vi "ReCalc_V2.00 - Kopie.vi"(3 "Berechnen":bool, 4 "Datenspeicher":T2={"Fahrzeugdaten"="", "date/time string"="", "Rolle [Inkr/U]"=0, "Rollenumfang [m]"=0.0, "Rollenträgheit [kgm²]"=0.0, "Zündung [Imp/U]"=0.0, "Getriebe [1:]"=0.0, "Reifenumfang [m] "=0.0, "element"=0.0, "Gl. Mittelwert"=0, "Differenzenquotient"=0, "Polynom"=0, "dT [s]"=0.0, "element"=0.0, "Lufttemperatur [°C]"=0.0, "Luftfeuchtigkeit [%]"=0.0, "Luftdruck [mbar]"=0.0, [], [], "Best Polynomial Fit"=[], [], "Übersetzung ermitteln aus"=0, "[s]"=0.0, "nmin [1/min]"=0.0, "nmax [1/min]"=0.0, "n vom Gas [1/min]"=0.0, "dT ungefiltert [s]"=[], [], "Boolesch"=FALSE, "Serielle Schnittstelle"="COM4", "nKuWe/nRolle 2"=10.0, "v vom Gas [km/h]"=5000.0}) -> ()   [LabVIEW 2014]
uses:
  <vilib>/Utility/miscctls.llb/LVPointTypeDef.ctl
  <vilib>/Analysis/3filter.llb/IIR Filter (DBL).vi
  <vilib>/Analysis/NI_AALBase.lvlib
  <vilib>/Utility/miscctls.llb/LVCursorListTypeDef.ctl
panel:
  in  "Rollenumfang [m] 2":dbl=0.613
  in  "v vom Gas [km/h]":dbl=5000.0
  in  "Legende":bool=TRUE
  out "Fahrzeugdaten":string
  out "Überlagerung":bool
  in  "Überlagern":bool
  out "Übersetzung ermitteln aus":T1(ring)
  in  "Speichern":bool
  out "Reifenumfang [m]":dbl=1.222
  out "Getriebe [1:]":dbl=5.343
  out "Zündung [Imp/U]":dbl=1.0
  out "Rollengeber [Inkr/U]":u16=200
  out "Luftdruck [mbar]":dbl=1013.0
  out "Luftfeuchtigkeit [%]":dbl=50.0
  out "Lufttemperatur [°C]":dbl=20.0
  in  "Stopp":bool
  in  "Rollenträgheit [kgm²]":dbl=0.402
  in  "Gl. Mittelwert":u8=35
  in  "Differenzenquotient":u8=12
  in  "n vom Gas [1/min]":dbl=5000.0
  out "Rollenumfang [m]":dbl=0.613 format="%.3f"
  out "Datum, Zeit":string
  out "Untersetzung aus:":dbl=2.68 format="%.2f"
  in  "Drucken":bool
  out "Pmax":string
  out "Ergebnis":string
  out "XY-Graph":cluster{dbl[], dbl[]}[](graph)
  in  "Öffnen":bool
  out "korr":dbl
  out "[s]":dbl=5.0
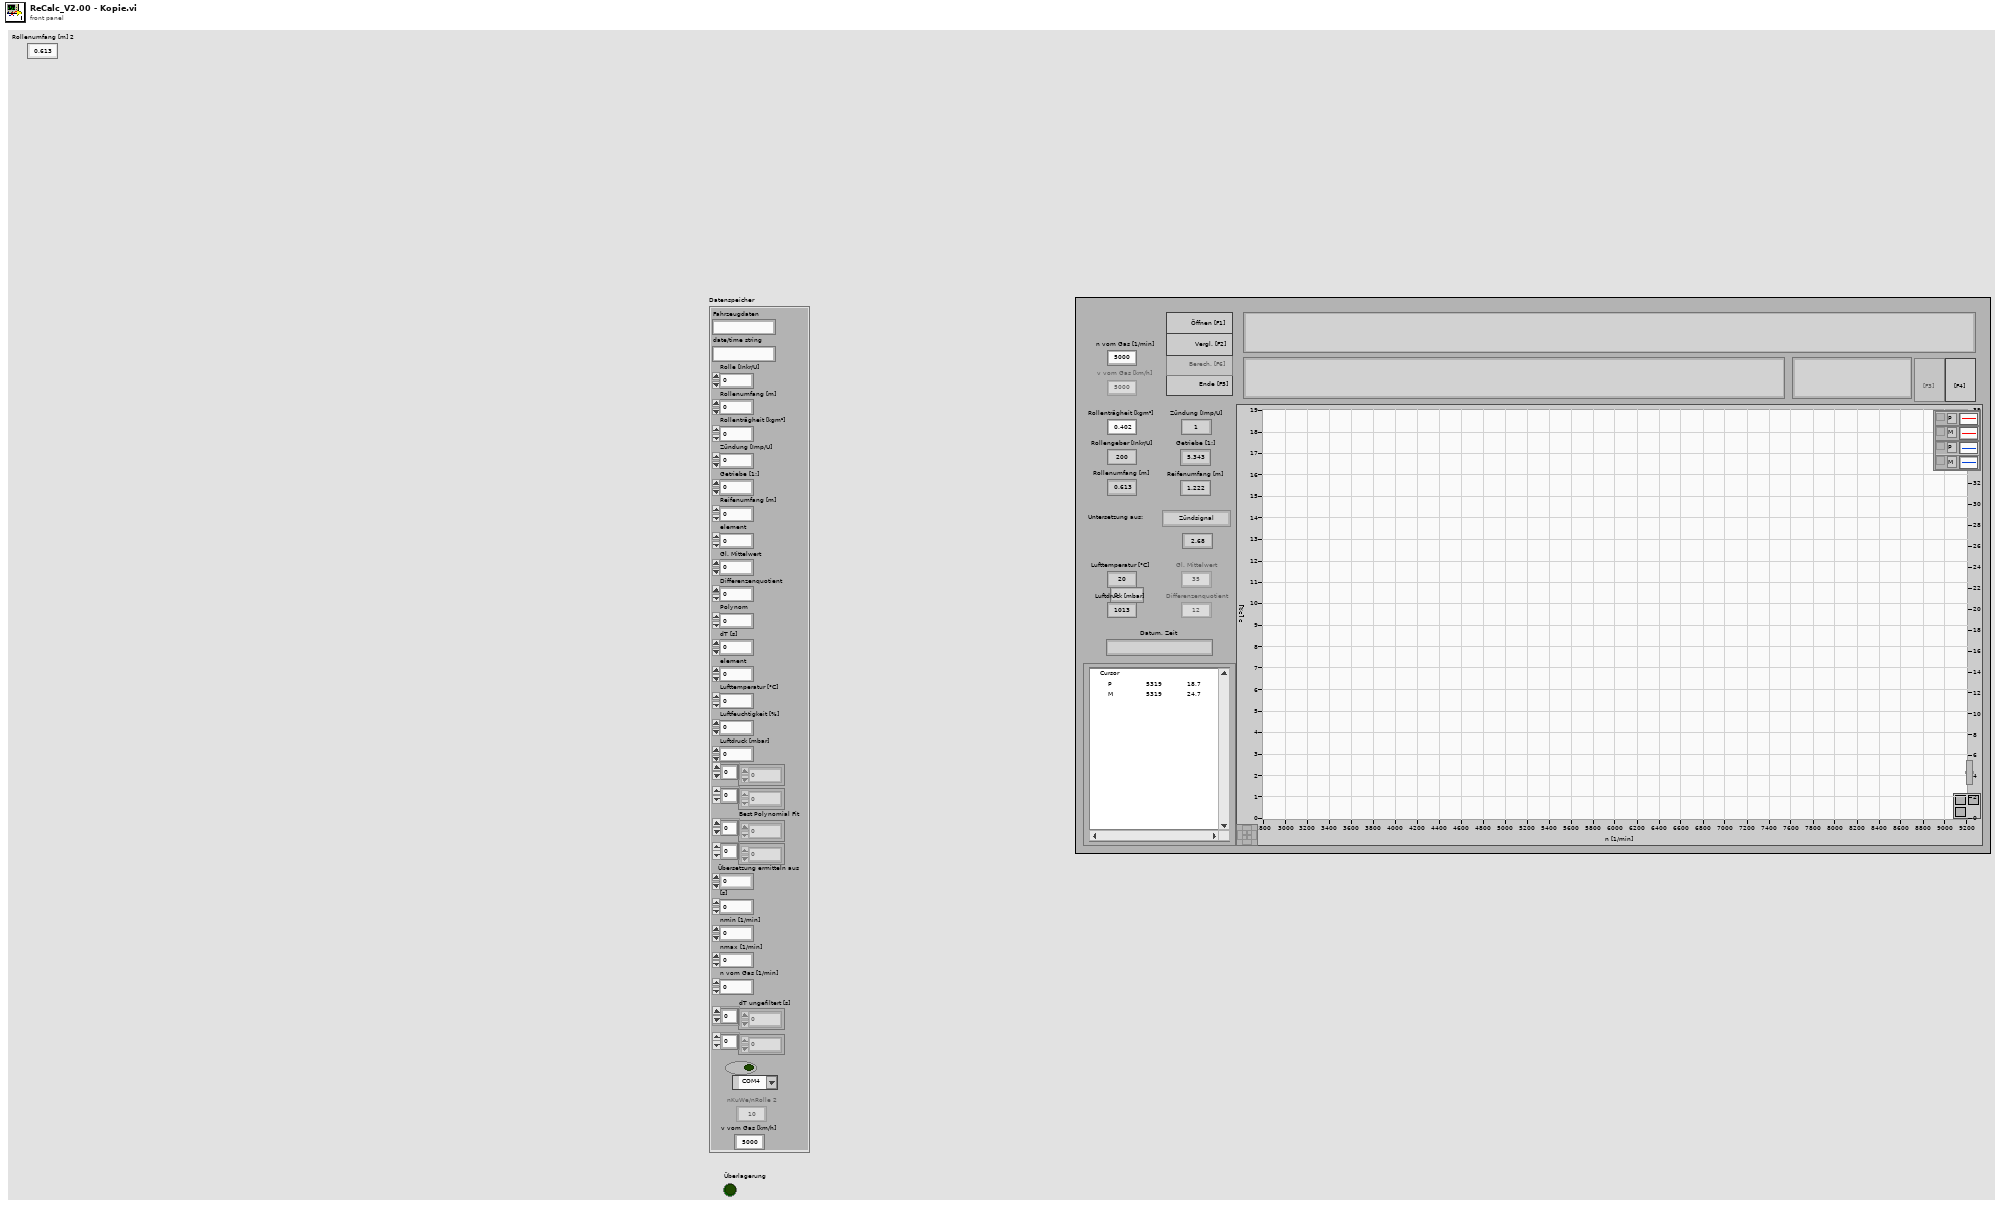
[diagram p1: front panel]
types:
  T1 = enum8{"Zündsignal", "Getriebe & Reifen", "nKuWe / nRolle", "Vario [km/h]"}
  T2 = cluster{"Fahrzeugdaten":string, "date/time string":string, "Rolle [Inkr/U]":u16, "Rollenumfang [m]":dbl, "Rollenträgheit [kgm²]":dbl, "Zündung [Imp/U]":dbl, "Getriebe [1:]":dbl, "Reifenumfang [m] ":dbl, "element":dbl, "Gl. Mittelwert":u8, "Differenzenquotient":u8, "Polynom":u8, "dT [s]":dbl, "element":dbl, "Lufttemperatur [°C]":dbl, "Luftfeuchtigkeit [%]":dbl, "Luftdruck [mbar]":dbl, dbl[], dbl[], "Best Polynomial Fit":dbl[], dbl[], "Übersetzung ermitteln aus":u8, "[s]":dbl, "nmin [1/min]":dbl, "nmax [1/min]":dbl, "n vom Gas [1/min]":dbl, "dT ungefiltert [s]":dbl[], i32[], "Boolesch":bool, "Serielle Schnittstelle":refnum<visa-resource-name>, "nKuWe/nRolle 2":dbl, "v vom Gas [km/h]":dbl}
  T3 = typedef "LVPointTypeDef.ctl" = cluster{"Horizontal":i16, "Vertical":i16}
  T4 = typedef "LVCursorListTypeDef.ctl" = cluster{"Name":string, "Color":u32, "Style":u8, "Point Style":u8, "Name Visible":bool, "Allow Drag":bool, "Cursor Mode":u32, "Plot":i32, "Index":i32, "Position":cluster{"X":dbl, "Y":dbl}, "X Scale":u32, "Y Scale":u32, "Watch Plots":i32[], "Watch All Plots":bool, "Plot Area":i32, "Label Offset":cluster{"X":dbl, "Y":dbl}}[]
  T5 = enum8{"Enabled", "Disabled", "Disabled and Grayed Out"}
  T6 = enum16{"Zündsignal", "Getriebe & Reifen", "nKuWe / nRolle", "Vario (km/h)"}
  T7 = cluster{"Fahrzeugdaten":string, "date/time string":string, "Rolle [Inkr/U]":u16, "Rollenumfang [m]":dbl, "Rollenträgheit [kgm²]":dbl, "Zündung [Imp/U]":dbl, "Getriebe [1:]":dbl, "Reifenumfang [m] ":dbl, "element":dbl, "Gl. Mittelwert":u8, "Differenzenquotient":u8, "Polynom":u8, "dT [s]":dbl, "element":dbl, "Lufttemperatur [°C]":dbl, "Luftfeuchtigkeit [%]":dbl, "Luftdruck [mbar]":dbl, dbl[], dbl[], "Best Polynomial Fit":dbl[], dbl[], "Übersetzung ermitteln aus":u8, "[s]":dbl, "nmin [1/min]":dbl, "nmax [1/min]":dbl, "n vom Gas [1/min]":dbl, "dT-Array [s]":dbl[], i32[], "Boolesch":bool, "Serielle Schnittstelle":refnum<visa-resource-name>, "nKuWe/nRolle":dbl, "v vom Gas [km/h]":dbl}
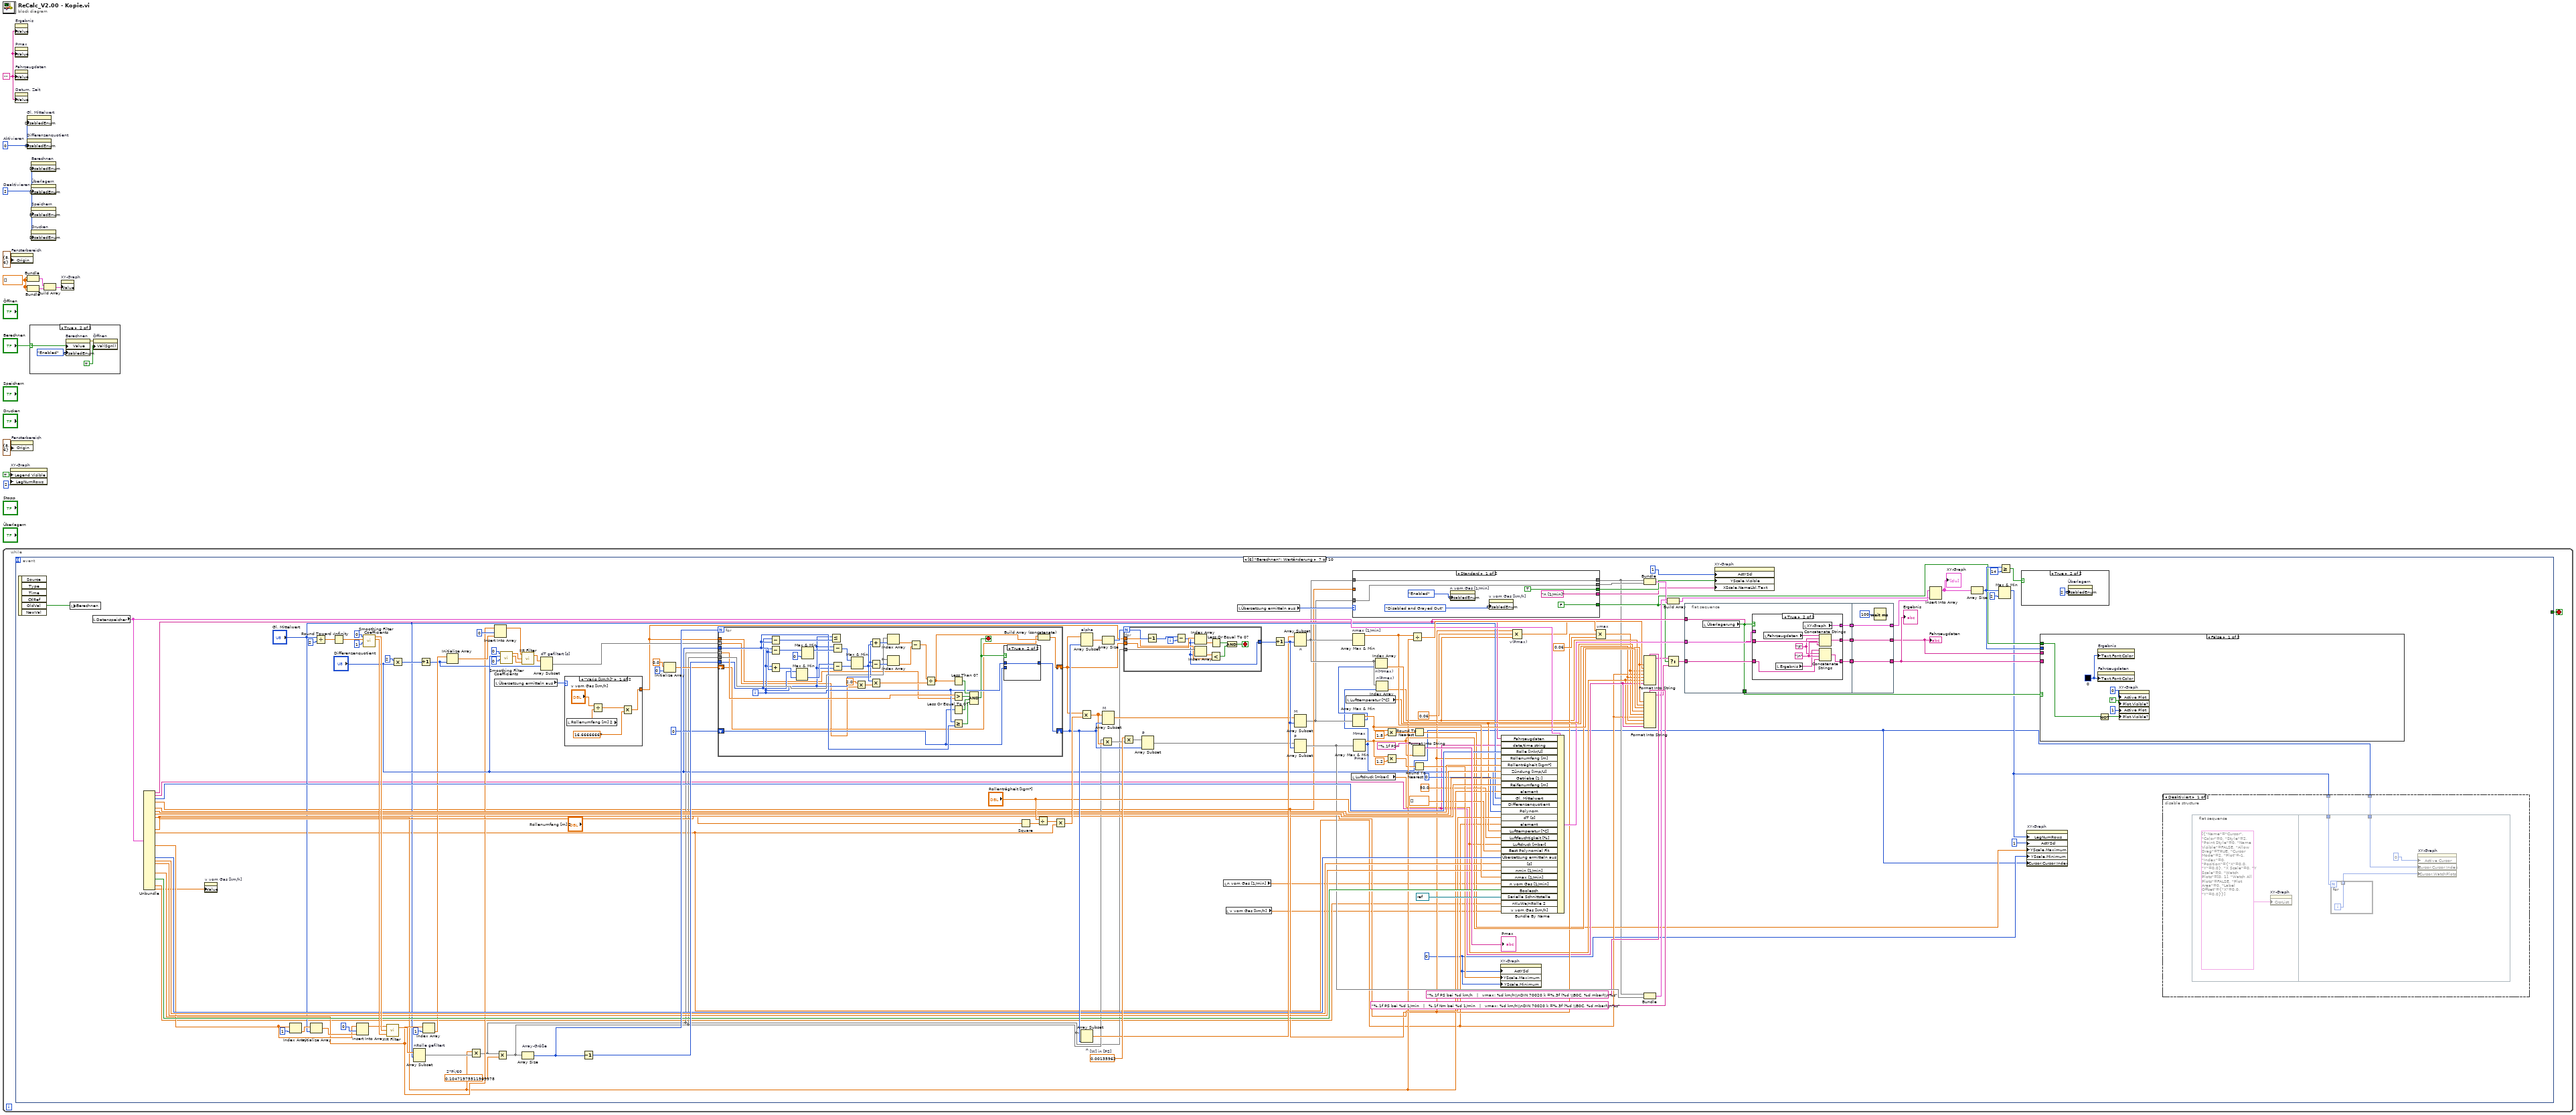
[diagram p0: block diagram]
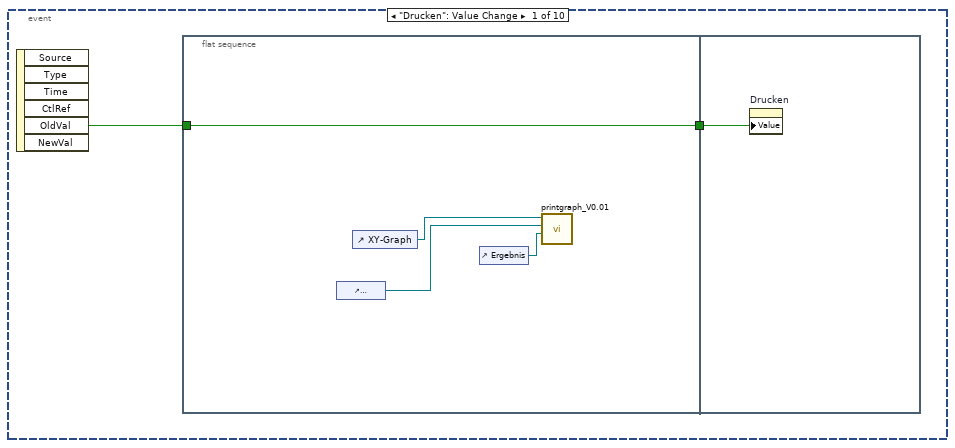
[diagram p3: hidden frame]
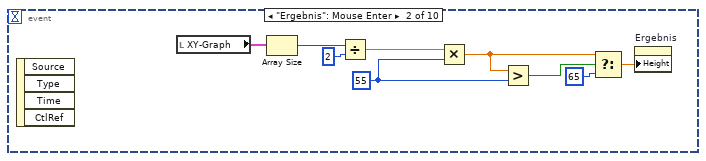
[diagram p4: hidden frame]
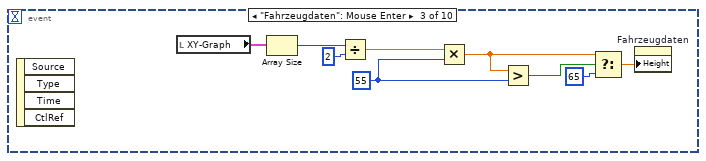
[diagram p5: hidden frame]
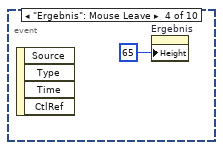
[diagram p6: hidden frame]
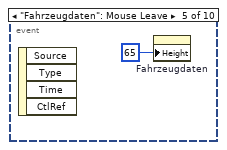
[diagram p7: hidden frame]
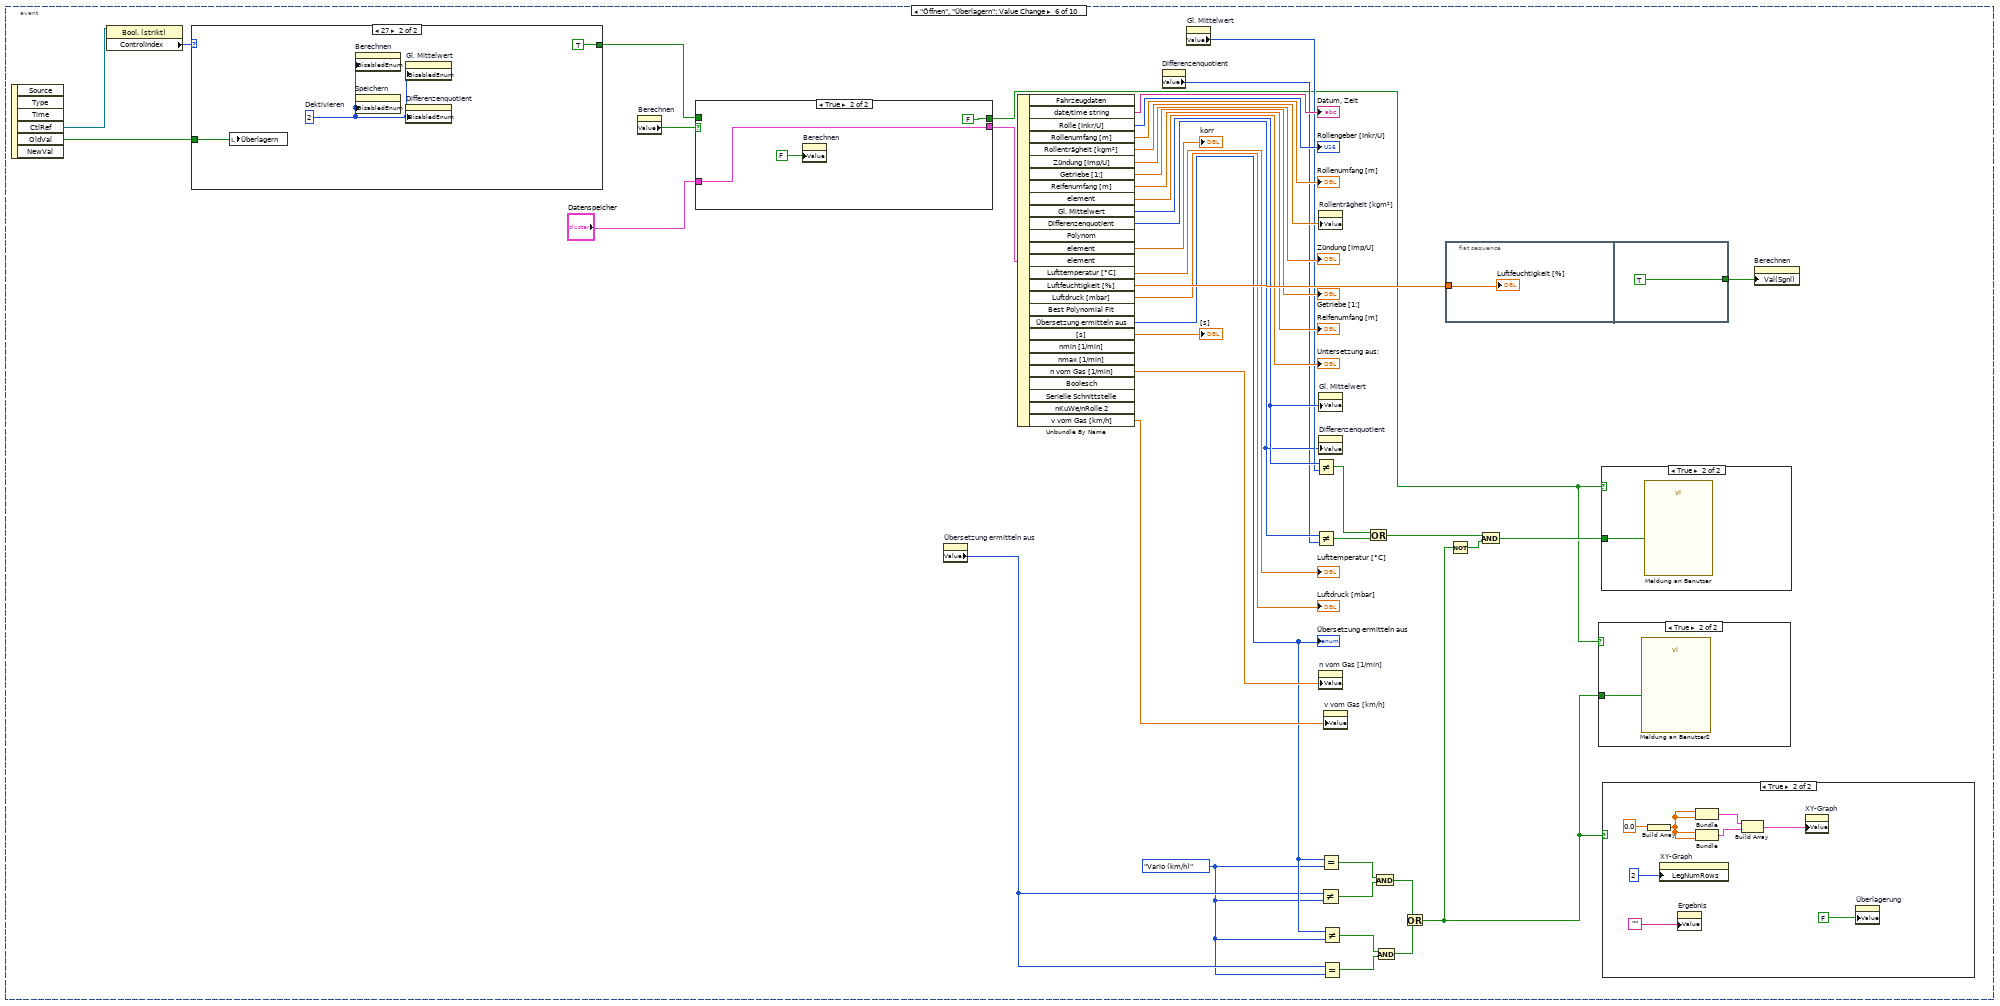
[diagram p8: hidden frame]
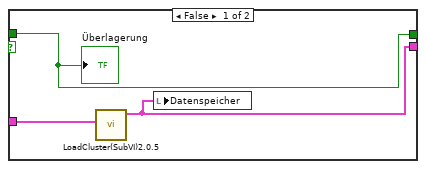
[diagram p12: hidden frame]
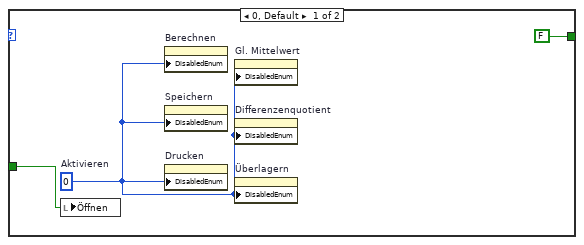
[diagram p13: hidden frame]
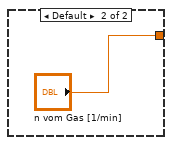
[diagram p15: hidden frame]
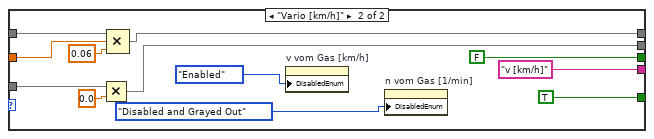
[diagram p16: hidden frame]
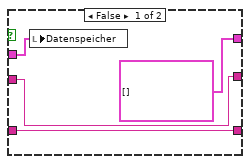
[diagram p18: hidden frame]
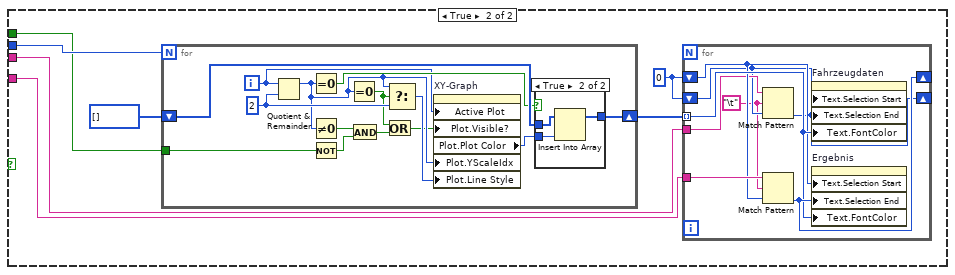
[diagram p19: hidden frame]
diagram:
  w2 = 0  # Aktivieren
  w8 = dbl[] []
  w4 = 2  # Deaktivieren
  w12 = ""
  n1 = while {
    stop <- w13 stop-if-true
    n2 = event shown="[6] \"Berechnen\": Wertänderung" {
      selector: _ -> [_ _ _ _ _ _ _ _ _ _]
      dyn-events: _ -> [_ _ _ _ _ _ _ _ _ _]
      timeout: _ -> [_ _ _ _ _ _ _ _ _ _]
      tunnel: [_ _ _ _ _ _ _ _ w396 _] -> w13
      event "Drucken": Value Change {
        n3 = event-data() -> ("OldVal"=w15:bool)  [unwired: 1 in, 5 out]
        n4 = flat-sequence {
          tunnel: [w19] -> w14
          tunnel: w15 -> [w19]
          tunnel: w14 -> [w20]
          frame #0 {
            n5 = control-ref of="Fahrzeugdaten"() -> (w17:refnum<vi>)
            n6 = control-ref of="XY-Graph"() -> (w18:refnum<vi>)
            n7 = control-ref of="Ergebnis"() -> (w16:refnum<vi>)
            n8 = call "printgraph_V0.01.vi"("reference 2"=w16, "Fahrzeugdaten"=w17, "XYGraph (Eingang)"=w18) -> ()  [unwired: 9 in]
          }
          frame #1 {
            n9 = property on="Drucken" class="Bool. (strikt)"("Value"=w20) -> ()  [unwired: 2 in, 2 out]
          }
        }
      }
      event "Ergebnis": Mouse Enter {
        w23 = u32 55 ("Größe:Höhe")
        n10 = event-data() -> ()  [unwired: 1 in, 4 out]
        n11 = local read "XY-Graph"() -> (w29:cluster{dbl[], dbl[]}[])
        n12 = Array Size(array=w29) -> (size(s)=w28:i32)
        n13 = Divide(x=w28, y=2) -> (x/y=w26:dbl)
        n14 = Multiply(x=w26, y=w23) -> (x*y=w24:dbl)
        n15 = Greater?(x=w24, y=w23) -> (0:w25:bool)
        n16 = Select(t=w24, s=w25, f=u32 65 ("Größe:Höhe")) -> (s? t:f=w22:dbl)
        n17 = property on="Ergebnis" class="Str"("Height"=w22) -> ()  [unwired: 2 in, 2 out]
      }
      event "Fahrzeugdaten": Mouse Enter {
        w32 = u32 55 ("Größe:Höhe")
        n18 = event-data() -> ()  [unwired: 1 in, 4 out]
        n19 = local read "XY-Graph"() -> (w38:cluster{dbl[], dbl[]}[])
        n20 = Array Size(array=w38) -> (size(s)=w37:i32)
        n21 = Divide(x=w37, y=2) -> (x/y=w35:dbl)
        n22 = Multiply(x=w35, y=w32) -> (x*y=w33:dbl)
        n23 = Greater?(x=w33, y=w32) -> (0:w34:bool)
        n24 = Select(t=w33, s=w34, f=u32 65 ("Größe:Höhe")) -> (s? t:f=w31:dbl)
        n25 = property on="Fahrzeugdaten" class="Str"("Height"=w31) -> ()  [unwired: 2 in, 2 out]
      }
      event "Ergebnis": Mouse Leave {
        n26 = event-data() -> ()  [unwired: 1 in, 4 out]
        n27 = property on="Ergebnis" class="Str"("Height"=u32 65 ("Größe:Höhe")) -> ()  [unwired: 2 in, 2 out]
      }
      event "Fahrzeugdaten": Mouse Leave {
        n28 = event-data() -> ()  [unwired: 1 in, 4 out]
        n29 = property on="Fahrzeugdaten" class="Str"("Height"=u32 65 ("Größe:Höhe")) -> ()  [unwired: 2 in, 2 out]
      }
      event "Öffnen", "Überlagern": Value Change {
        w51 = T6."Vario (km/h)"
        n30 = event-data() -> ("CtlRef"=w82:refnum<vi>, "OldVal"=w80:bool)  [unwired: 1 in, 4 out]
        n31 = property class="Bool. (strikt)"(reference=w82) -> ("ControlIndex"=w81:i32)  [unwired: 1 in, 2 out]
        n32 = case shown="27" w81 {
          tunnel: w80 -> [w104 w107]
          tunnel: [FALSE ("Überlagerung") TRUE ("Überlagerung")] -> w79
          frame 0, Default {
            w102 = 0  # Aktivieren
            n33 = local write "Öffnen"(w104) -> ()
            n34 = property on="Berechnen" class="Bool. (strikt)"("DisabledEnum"=w102) -> ()  [unwired: 2 in, 2 out]
            n35 = property on="Speichern" class="Bool. (strikt)"("DisabledEnum"=w102) -> ()  [unwired: 2 in, 2 out]
            n36 = property on="Drucken" class="Bool. (strikt)"("DisabledEnum"=w102) -> ()  [unwired: 2 in, 2 out]
            n37 = property on="Gl. Mittelwert" class="DigWert (strikt)"("DisabledEnum"=w102) -> ()  [unwired: 2 in, 2 out]
            n38 = property on="Differenzenquotient" class="DigWert (strikt)"("DisabledEnum"=w102) -> ()  [unwired: 2 in, 2 out]
            n39 = property on="Überlagern" class="Bool. (strikt)"("DisabledEnum"=w102) -> ()  [unwired: 2 in, 2 out]
          }
          frame 27 {
            w105 = 2  # Dektivieren
            n40 = local write "Überlagern"(w107) -> ()
            n41 = property on="Berechnen" class="Bool. (strikt)"("DisabledEnum"=w105) -> ()  [unwired: 2 in, 2 out]
            n42 = property on="Speichern" class="Bool. (strikt)"("DisabledEnum"=w105) -> ()  [unwired: 2 in, 2 out]
            n43 = property on="Gl. Mittelwert" class="DigWert (strikt)"("DisabledEnum"=w105) -> ()  [unwired: 2 in, 2 out]
            n44 = property on="Differenzenquotient" class="DigWert (strikt)"("DisabledEnum"=w105) -> ()  [unwired: 2 in, 2 out]
          }
        }
        n45 = property on="Berechnen" class="Bool. (strikt)"() -> ("Value"=w64:bool)  [unwired: 2 in, 2 out]
        n46 = case shown="True" w64 {
          tunnel: "Datenspeicher" -> [w95 w98]
          tunnel: w79 -> [w96 _]
          tunnel: [w94 w98] -> w65
          tunnel: [w96 FALSE] -> w42
          frame False {
            n47 = call "LoadCluster(SubVI)2.0.5.vi"("Datenspeicher"=w95) -> ("Value"=w94:T7)  [unwired: 10 in]
            n48 = local write "Datenspeicher"(w94) -> ()
            "Überlagerung" <- w96
          }
          frame True {
            n49 = property on="Berechnen" class="Bool. (strikt)"("Value"=FALSE) -> ()  [unwired: 2 in, 2 out]
          }
        }
        n50 = property on="Übersetzung ermitteln aus" class="Enum (strikt)"() -> ("Value"=w52:T1)  [unwired: 2 in, 2 out]
        n51 = Unbundle By Name(w65) -> ("date/time string"=→"Datum, Zeit":string, "Rolle [Inkr/U]"=→"Rollengeber [Inkr/U]":u16, "Rollenumfang [m]"=→"Rollenumfang [m]":dbl, "Rollenträgheit [kgm²]"=w69:dbl, "Zündung [Imp/U]"=→"Zündung [Imp/U]":dbl, "Getriebe [1:]"=→"Getriebe [1:]":dbl, "Reifenumfang [m]"=→"Reifenumfang [m]":dbl, "element"=→"Untersetzung aus:":dbl, "Gl. Mittelwert"=w63:u8, "Differenzenquotient"=w61:u8, "element"=→"korr":dbl, "Lufttemperatur [°C]"=→"Lufttemperatur [°C]":dbl, "Luftfeuchtigkeit [%]"=w76:dbl, "Luftdruck [mbar]"=→"Luftdruck [mbar]":dbl, "Übersetzung ermitteln aus"=w53:u8, "[s]"=→"[s]":dbl, "n vom Gas [1/min]"=w78:dbl, "v vom Gas [km/h]"=w56:dbl)  [unwired: 9 out]
        "Übersetzung ermitteln aus" <- w53
        n52 = property on="Differenzenquotient" class="DigWert (strikt)"() -> ("Value"=w60:u8)  [unwired: 2 in, 2 out]
        n53 = property on="Gl. Mittelwert" class="DigWert (strikt)"() -> ("Value"=w62:u8)  [unwired: 2 in, 2 out]
        n54 = Not Equal?(x=w63, y=w62) -> (x != y?=w59:bool)
        n55 = Not Equal?(x=w61, y=w60) -> (x != y?=w58:bool)
        n56 = property on="Rollenträgheit [kgm²]" class="DigWert (strikt)"("Value"=w69) -> ()  [unwired: 2 in, 2 out]
        n57 = property on="Gl. Mittelwert" class="DigWert (strikt)"("Value"=w63) -> ()  [unwired: 2 in, 2 out]
        n58 = property on="Differenzenquotient" class="DigWert (strikt)"("Value"=w61) -> ()  [unwired: 2 in, 2 out]
        n59 = property on="n vom Gas [1/min]" class="DigWert (strikt)"("Value"=w78) -> ()  [unwired: 2 in, 2 out]
        n60 = Not Equal?(x=w52, y=w51) -> (x != y?=w54:bool)
        n61 = Equal?(x=w53, y=w51) -> (x = y?=w55:bool)
        n62 = Not Equal?(x=w53, y=w51) -> (x != y?=w50:bool)
        n63 = Equal?(x=w52, y=w51) -> (x = y?=w49:bool)
        n64 = property on="v vom Gas [km/h]" class="DigWert (strikt)"("Value"=w56) -> ()  [unwired: 2 in, 2 out]
        n65 = Or(x=w59, y=w58) -> (x .or. y?=w44:bool)
        n66 = And(x=w55, y=w54) -> (x .and. y?=w48:bool)
        n67 = And(x=w50, y=w49) -> (x .and. y?=w47:bool)
        n68 = Or(x=w48, y=w47) -> (x .or. y?=w41:bool)
        n69 = flat-sequence {
          tunnel: w76 -> [w100]
          tunnel: [TRUE] -> w43
          frame #0 {
            "Luftfeuchtigkeit [%]" <- w100
          }
          frame #1 {
          }
        }
        n70 = Not(x=w41) -> (.not. x?=w45:bool)
        n71 = And(x=w44, y=w45) -> (x .and. y?=w46:bool)
        n72 = case shown="True" w42 {
          tunnel: w41 -> [_ w92]
          frame False {
          }
          frame True {
            n73 = call "Meldung an Benutzer2"("Enable"=w92) -> ()  [unwired: 9 in, 2 out]
          }
        }
        n74 = case shown="True" w42 {
          tunnel: w46 -> [_ w93]
          frame False {
          }
          frame True {
            n75 = call "Meldung an Benutzer"("Enable"=w93) -> ()  [unwired: 9 in, 2 out]
          }
        }
        n76 = case shown="True" w41 {
          frame False {
          }
          frame True {
            n77 = Build Array(0.0) -> (w91:dbl[])
            n78 = property on="XY-Graph" class="XYGraph (strikt)"("LegNumRows"=2) -> ()  [unwired: 2 in, 2 out]
            n79 = property on="Ergebnis" class="Str"("Value"="") -> ()  [unwired: 2 in, 2 out]
            n80 = Bundle(w91, w91) -> (w87:cluster{dbl[], dbl[]})  [unwired: 1 in]
            n81 = Bundle(w91, w91) -> (w88:cluster{dbl[], dbl[]})  [unwired: 1 in]
            n82 = Build Array(w87, w88) -> (w89:cluster{dbl[], dbl[]}[])
            n83 = property on="XY-Graph" class="XYGraph (strikt)"("Value"=w89) -> ()  [unwired: 2 in, 2 out]
            n84 = property on="Überlagerung" class="Bool. (strikt)"("Value"=FALSE) -> ()  [unwired: 2 in, 2 out]
          }
        }
        n85 = property on="Berechnen" class="Bool. (strikt)"("Val(Sgnl)"=w43) -> ()  [unwired: 2 in, 2 out]
      }
      event "Berechnen": Value Change {
        w113 = 0
        w235 = 0.00135962  # [W] in [PS]
        w242 = 0.10471975511965978  # 2*Pi/60
        n86 = event-data() -> ("OldVal"=w194:bool)  [unwired: 1 in, 5 out]
        n87 = local write "Berechnen"(w194) -> ()
        n88 = local read "Datenspeicher"() -> (w206:T2)
        n89 = Unbundle(w206) -> ("Fahrzeugdaten"=w186:string, "date/time string"=w134:string, "Rolle [Inkr/U]"=w205:u16, "Rollenumfang [m]"=w137:dbl, "Zündung [Imp/U]"=w200:dbl, "Getriebe [1:]"=w199:dbl, "Reifenumfang [m]"=w198:dbl, "element"=w150:dbl, "dT [s]"=w160:dbl, "element"=w131:dbl, w159:dbl[], "Übersetzung ermitteln aus"=w201:u8, "[s]"=w195:dbl, "nmin [1/min]"=w196:dbl, "dT ungefiltert [s]"=w158:dbl[], "Boolesch"=w203:bool, "nKuWe/nRolle 2"=w121:dbl, "v vom Gas [km/h]"=w118:dbl)  [unwired: 14 out]
        n90 = property on="v vom Gas [km/h]" class="DigWert (strikt)"("Value"=w118) -> ()  [unwired: 2 in, 2 out]
        n91 = Index Array(array=w159, index=1) -> (element=w211:dbl)
        n92 = Initialize Array(w211, "Gl. Mittelwert") -> (w212:dbl[])
        n93 = Divide(x="Gl. Mittelwert", y=2) -> (x/y=w245:dbl)
        n94 = Round Toward -Infinity(1:w245) -> (0:w244:dbl)
        n95 = Insert Into Array ("In Array einfügen")(array=w159, index=0, new element=w212) -> (w209:dbl[])
        n96 = call <vilib>:"Smoothing Filter Coefficients.vi"("shape"=1, "half-width"=w244, "type"=0) -> ("forward coefficients"=w213:dbl[], "reverse coefficients"=w214:dbl[])  [unwired: 6 in, 1 out]
        n97 = call-poly <vilib>:"IIR Filter.vi"("Forward Coefficients"=w213, "Reverse Coefficients"=w214, "X"=w209) -> ("Filtered X"=w208:dbl[])  [unwired: 1 in, 1 out]
        n98 = Multiply(x=2, y="Differenzenquotient") -> (x*y=w168:i32)
        n99 = Array Subset "nRolle gefiltert"(array=w208, index="Gl. Mittelwert") -> (w152:dbl[])  [unwired: 1 in]
        n100 = Increment(x=w168) -> (x+1=w161:i32)
        n101 = Index Array(array=w158, index=1 ("Index")) -> (element=w166:dbl)
        n102 = Initialize Array(w166, w161) -> (w164:dbl[])
        n103 = Multiply(x=w150, y=w152) -> (x*y=w151:dbl[])
        n104 = Insert Into Array(array=w158, index=0 ("Index"), new element=w164) -> (w163:dbl[])
        n105 = local read "Übersetzung ermitteln aus"() -> (w116:T1)
        n106 = Multiply(x=w151, y=w242) -> (x*y=w154:dbl[])
        n107 = call <vilib>:"Smoothing Filter Coefficients.vi"("shape"=0, "half-width"="Differenzenquotient", "type"=0) -> ("forward coefficients"=w171:dbl[], "reverse coefficients"=w172:dbl[])  [unwired: 6 in, 1 out]
        n108 = call-poly <vilib>:"IIR Filter.vi"("Forward Coefficients"=w171, "Reverse Coefficients"=w172, "X"=w163) -> ("Filtered X"=w162:dbl[])  [unwired: 1 in, 1 out]
        n109 = Array Size "Array-Größe"(array=w154) -> (size(s)=w240:i32)
        n110 = Array Subset "dT gefiltert [s]"(array=w162, index=w161) -> (w153:dbl[])  [unwired: 1 in]
        n111 = case shown="\"Vario [km/h]\"" w116 {
          tunnel: [w259 "n vom Gas [1/min]"] -> w117
          frame "Vario [km/h]" {
            n112 = local read "Rollenumfang [m] 2"() -> (w260:dbl)
            n113 = Divide(x="v vom Gas [km/h]", y=w260) -> (x/y=w258:dbl)
            n114 = Multiply(x=w258, y=16.66666667) -> (x*y=w259:dbl)
          }
          frame Default {
          }
        }
        n115 = Decrement(x=w240) -> (x-1=w241:i32)
        n116 = Initialize Array(0.0 ("y"), 0) -> (w237:dbl[])
        n117 = for {
          N: w240 -> [_]
          tunnel: "Differenzenquotient" -> [w371]
          tunnel: w154 -> [w377]
          tunnel: w241 -> [w370]
          shift-right: [w375] -> w155
          shift-left: w237 -> [w358]
          tunnel: w151 -> [w373] mode=indexing
          tunnel: w117 -> [w362]
          shift-right: [w361] -> w228
          shift-left: 0 -> [w364]
          tunnel: w153 -> [w357] mode=indexing
          i -> [w365]
          stop <- w363 stop-if-true
          n118 = Subtract(x=w370, y=w371) -> (x-y=w372:i32)
          n119 = Subtract(x=w365, y=w371) -> (x-y=w390:i32)
          n120 = Add(x=w365, y=w371) -> (x+y=w384:i32)
          n121 = Max & Min(x=w370, y=w384) -> (min(x,y)=w385:i32)  [unwired: 1 out]
          n122 = Max & Min(x=w390, y=0) -> (max(x,y)=w388:i32)  [unwired: 1 out]
          n123 = Less Or Equal?(x=w365, y=w372) -> ()  [unwired: 1 out]
          n124 = Subtract(x=w365, y=w388) -> (x-y=w387:i32)
          n125 = Subtract(x=w385, y=w365) -> (x-y=w386:i32)
          n126 = Max & Min(x=w387, y=w386) -> (min(x,y)=w378:i32)  [unwired: 1 out]
          n127 = Multiply(x=2.0, y=w357) -> (x*y=w359:dbl)
          n128 = Add(x=w365, y=w378) -> (x+y=w383:i32)
          n129 = Subtract(x=w365, y=w378) -> (x-y=w382:i32)
          n130 = Multiply(x=w378, y=w359) -> (x*y=w376:dbl)
          n131 = Index Array(array=w377, index=w383) -> (element=w380:dbl)
          n132 = Index Array(array=w377, index=w382) -> (element=w381:dbl)
          n133 = Subtract(x=w380, y=w381) -> (x-y=w379:dbl)
          n134 = Divide(x=w379, y=w376) -> (x/y=w369:dbl)
          n135 = Less Than 0?(x=w369) -> (x < 0?=w367:bool)
          n136 = Greater?(x=w373, y=w362) -> (0:w374:bool)
          n137 = Less Or Equal To 0?(x=w364) -> (x <= 0?=w366:bool)
          n138 = Greater Or Equal?(x=w365, y=w371) -> (x >= y?=w368:bool)
          n139 = Compound Arithmetic op=AND(w367, w374, w366, w368) -> (w363:bool)
          n140 = case shown="True" w363 {
            tunnel: w365 -> [_ w392]
            tunnel: [w391 w392] -> w361
            tunnel: w364 -> [w391 _]
            frame False {
            }
            frame True {
            }
          }
          n141 = Build Array (concatenate)(w358, w369) -> (w375:dbl[])
        }
        n142 = Square(x=w150) -> (x^2=w236:dbl)
        n143 = Divide(x="Rollenträgheit [kgm²]", y=w236) -> (x/y=w233:dbl)
        n144 = Multiply(x=w233, y=w131) -> (x*y=w232:dbl)
        n145 = Multiply(x=w155, y=w232) -> (x*y=w217:dbl[])
        n146 = Array Subset "alpha"(array=w155, length=w228) -> (w230:dbl[])  [unwired: 1 in]
        n147 = Array Subset "n"(array=w151, length=w228) -> (w215:dbl[])  [unwired: 1 in]
        n148 = Multiply(x=w154, y=w217) -> (x*y=w234:dbl[])
        n149 = Array Size(array=w230) -> (size(s)=w227:i32)
        n150 = Array Subset "M"(array=w217, length=w228) -> (w157:dbl[])  [unwired: 1 in]
        n151 = Multiply(x=w235, y=w234) -> (x*y=w229:dbl[])
        n152 = for {
          N: w227 -> [w356]
          tunnel: w155 -> [w353]
          tunnel: w151 -> [w350]
          tunnel: w117 -> [w347]
          tunnel: [w345] -> w226
          i -> [w351]
          stop <- w346 stop-if-true
          n153 = Decrement(x=w356) -> (x-1=w355:i32)
          n154 = Subtract(x=w355, y=w351) -> (x-y=w345:i32)
          n155 = Index Array(array=w353, index=w345) -> (element=w354:dbl)
          n156 = Index Array(array=w350, index=w345) -> (element=w349:dbl)
          n157 = Less?(x=w349, y=w347) -> (x < y?=w348:bool)
          n158 = Less Or Equal To 0?(x=w354) -> (x <= 0?=w352:bool)
          n159 = And(x=w352, y=w348) -> (x .and. y?=w346:bool)
        }
        n160 = Array Subset "P"(array=w229, length=w228) -> (w156:dbl[])  [unwired: 1 in]
        n161 = local read "n vom Gas [1/min]"() -> (w120:dbl)
        n162 = local read "v vom Gas [km/h]"() -> (w119:dbl)
        n163 = local read "Übersetzung ermitteln aus"() -> (w142:T1)
        n164 = Increment(x=w226) -> (x+1=w225:i32)
        n165 = Array Subset "M"(array=w157, index=w225) -> (w122:dbl[])  [unwired: 1 in]
        n166 = Array Subset "P"(array=w156, index=w225) -> (w178:dbl[])  [unwired: 1 in]
        n167 = Array Subset "n"(array=w215, index=w225) -> (w141:dbl[])  [unwired: 1 in]
        n168 = local read "Lufttemperatur [°C]"() -> (w132:dbl)
        n169 = local read "Luftdruck [mbar]"() -> (w133:dbl)
        n170 = case shown="Standard" w142 {
          tunnel: w137 -> [_ w279]
          tunnel: w141 -> [w268 w278]
          tunnel: [w268 w271] -> w111
          tunnel: [FALSE TRUE] -> w123
          tunnel: [TRUE FALSE] -> w125
          tunnel: ["n [1/min]" "v [km/h]"] -> w124
          tunnel: w122 -> [w264 w274]
          tunnel: [w264 w272] -> w112
          frame Default {
            n171 = property on="n vom Gas [1/min]" class="DigWert (strikt)"("DisabledEnum"=T5."Enabled" ("Deaktiviert")) -> ()  [unwired: 2 in, 2 out]
            n172 = property on="v vom Gas [km/h]" class="DigWert (strikt)"("DisabledEnum"=T5."Disabled and Grayed Out" ("Deaktiviert")) -> ()  [unwired: 2 in, 2 out]
          }
          frame "Vario [km/h]" {
            n173 = Multiply(x=w274, y=0.0) -> (x*y=w272:dbl[])
            n174 = Compound Arithmetic op=MULTIPLY(w278, w279, 0.06) -> (w271:dbl[])
            n175 = property on="v vom Gas [km/h]" class="DigWert (strikt)"("DisabledEnum"=T5."Enabled" ("Deaktiviert")) -> ()  [unwired: 2 in, 2 out]
            n176 = property on="n vom Gas [1/min]" class="DigWert (strikt)"("DisabledEnum"=T5."Disabled and Grayed Out" ("Deaktiviert")) -> ()  [unwired: 2 in, 2 out]
          }
        }
        n177 = Array Max & Min "nmax [1/min]"(array=w141) -> (max value=w197:dbl)  [unwired: 3 out]
        n178 = Array Max & Min "Mmax"(array=w122) -> (max value=w219:dbl, max index (indices)=w110:i32)  [unwired: 2 out]
        n179 = Array Max & Min "Pmax"(array=w178) -> (max value=w139:dbl, max index (indices)=w108:i32)  [unwired: 2 out]
        n180 = Index Array "n(Mmax)"(array=w141, index=w110) -> (element=w202:dbl)
        n181 = Index Array "n(Pmax)"(array=w141, index=w108) -> (element=w135:dbl)
        n182 = Multiply(x=w219, y=1.8) -> (x*y=w149:dbl)
        n183 = Multiply(x=w139, y=1.2) -> (x*y=w147:dbl)
        n184 = Divide(x=w197, y=w150) -> (x/y=w222:dbl)
        n185 = Format Into String(format string="%.1f PS" ("Format-String"), w139) -> (resulting string=→"Pmax":string)  [unwired: 2 in, 1 out]
        n186 = Round To Nearest(number=w149) -> (nearest integer value=w114:dbl)
        n187 = Round To Nearest(number=w147) -> (nearest integer value=w148:dbl)
        n188 = property on="XY-Graph" class="XYGraph (strikt)"("ActYScl"=w113, "YScale.Maximum"=w148, "YScale.Minimum"=w113) -> ()  [unwired: 2 in, 2 out]
        n189 = Bundle By Name(cluster=w206, "Fahrzeugdaten"=w186, "date/time string"=w134, "Rolle [Inkr/U]"=w205, "Rollenumfang [m]"=w137, "Rollenträgheit [kgm²]"="Rollenträgheit [kgm²]", "Zündung [Imp/U]"=w200, "Getriebe [1:]"=w199, "Reifenumfang [m]"=w198, "element"=w150, "Gl. Mittelwert"="Gl. Mittelwert", "Differenzenquotient"="Differenzenquotient", "Polynom"=0, "dT [s]"=w160, "element"=w131, "Lufttemperatur [°C]"=w132, "Luftfeuchtigkeit [%]"=50.0, "Luftdruck [mbar]"=w133, "Best Polynomial Fit"=dbl[] [], "Übersetzung ermitteln aus"=w201, "[s]"=w195, "nmin [1/min]"=w196, "nmax [1/min]"=w197, "n vom Gas [1/min]"=w120, "Boolesch"=w203, "Serielle Schnittstelle"=refnum<visa-resource-name> refnum, "nKuWe/nRolle 2"=w121, "v vom Gas [km/h]"=w119) -> (w192:T2)
        n190 = Compound Arithmetic op=MULTIPLY "v(Pmax)"(w137, 0.06, w135) -> (w138:dbl)
        n191 = Compound Arithmetic op=MULTIPLY "vmax"(w222, w137, 0.06) -> (w130:dbl)
        n192 = Bundle(w111, w112) -> (w180:cluster{dbl[], dbl[]})  [unwired: 1 in]
        n193 = Format Into String(format string="%.1f PS bei %d km/h   |   vmax: %d km/h\\nDIN 70020 k =%.3f (%d \\B0C, %d mbar)\\n%s" ("Format-String"), w139, w138, w130, w131, w132, w133, w134) -> (resulting string=w127:string)  [unwired: 2 in, 1 out]
        n194 = Format Into String(format string="%.1f PS bei %d 1/min   |   %.1f Nm bei %d 1/min   |   vmax: %d km/h\\nDIN 70020 k =%.3f (%d \\B0C, %d mbar)\\n%s" ("Format-String"), w139, w135, w219, w202, w130, w131, w132, w133, w134) -> (resulting string=w128:string)  [unwired: 2 in, 1 out]
        n195 = Bundle(w111, w178) -> (w181:cluster{dbl[], dbl[]})  [unwired: 1 in]
        n196 = Build Array(w181, w180) -> (w190:cluster{dbl[], dbl[]}[])
        n197 = Select(t=w127, s=w123, f=w128) -> (s? t:f=w129:string)
        n198 = flat-sequence {
          tunnel: w129 -> [w288]
          tunnel: w192 -> [w287]
          tunnel: [w286] -> w191
          tunnel: w186 -> [w282]
          tunnel: [w285] -> w185
          tunnel: [w284] -> w184
          tunnel: [w283] -> w183
          tunnel: [w303] -> w187
          tunnel: [w304] -> w188
          tunnel: [w305] -> w189
          tunnel: w185 -> [w305]
          tunnel: w184 -> [w304]
          tunnel: w183 -> [w303]
          frame #0 {
            n199 = local read "Überlagerung"() -> (w286:bool)
            n200 = case shown="True" w286 {
              tunnel: [cluster{dbl[], dbl[]}[] [] ("XY-Graph") w301] -> w285
              tunnel: w288 -> [w291 w299]
              tunnel: [w291 w300] -> w284
              tunnel: w287 -> [w290 _]
              tunnel: w282 -> [w289 w297]
              tunnel: [w289 w296] -> w283
              frame False {
                n201 = local write "Datenspeicher"(w290) -> ()
              }
              frame True {
                w295 = "\t"
                w298 = "\n"
                n202 = local read "Fahrzeugdaten"() -> (w294:string)
                n203 = local read "Ergebnis"() -> (w293:string)
                n204 = local read "XY-Graph"() -> (w301:cluster{dbl[], dbl[]}[])
                n205 = Concatenate Strings(w294, w295, w298, w297) -> (w296:string)
                n206 = Concatenate Strings(w293, w295, w298, w299) -> (w300:string)
              }
            }
          }
          frame #1 {
            n207 = Wait (ms)(milliseconds to wait=u32 100 ("Zu wartende ms")) -> ()  [unwired: 1 out]
          }
        }
        n208 = property on="XY-Graph" class="XYGraph (strikt)"("ActYScl"=1, "YScale.Visible"=w125, "XScale.NameLbl.Text"=w124) -> ()  [unwired: 2 in, 2 out]
        n209 = Insert Into Array(array=w189, new element=w190) -> (w193:cluster{dbl[], dbl[]}[])  [unwired: 1 in]
        "XY-Graph" <- w193
        n210 = Array Size(array=w193) -> (size(s)=w145:i32)
        n211 = Max & Min(x=w145, y=2) -> (max(x,y)=w109:i32)  [unwired: 1 out]
        n212 = Greater Or Equal?(x=w145, y=14) -> (x >= y?=w175:bool)
        n213 = case shown="True" w175 {
          frame False {
          }
          frame True {
            n214 = property on="Überlagern" class="Bool. (strikt)"("DisabledEnum"=2) -> ()  [unwired: 2 in, 2 out]
          }
        }
        n215 = property on="XY-Graph" class="XYGraph (strikt)"("LegNumRows"=w109, "ActYScl"=1, "YScale.Maximum"=w114, "YScale.Minimum"=w113, "Cursor.Cursor Index"=w108) -> ()  [unwired: 2 in, 2 out]
        n216 = case shown="False" w191 {
          tunnel: w145 -> [_ w318]
          tunnel: w188 -> [_ w315]
          tunnel: w187 -> [_ w314]
          tunnel: w123 -> [w306 w312]
          frame False {
            w311 = u32 0
            n217 = property on="Ergebnis" class="Str"("Text.Font:Color"=w311) -> ()  [unwired: 2 in, 2 out]
            n218 = property on="Fahrzeugdaten" class="Str"("Text.Font:Color"=w311) -> ()  [unwired: 2 in, 2 out]
            n219 = Not(x=w306) -> (.not. x?=w307:bool)
            n220 = property on="XY-Graph" class="XYGraph (strikt)"("Active Plot"=0, "Plot.Visible?"=TRUE ("Plot.Sichtbar"), "Active Plot"=1, "Plot.Visible?"=w307) -> ()  [unwired: 2 in, 2 out]
          }
          frame True {
            w313 = 0
            n221 = for {
              N: w318 -> [_]
              shift-right: [w340] -> w316
              shift-left: u32[] [] -> [w339]
              tunnel: w312 -> [w332]
              i -> [w334]
              w337 = 2 ("y")
              n222 = Quotient & Remainder(x=w334, y=w337) -> (x-y*floor(x/y)=w333:i32)  [unwired: 1 out]
              n223 = Equal To 0?(x=w333) -> (x = 0?=w338:bool)
              n224 = Not Equal To 0?(x=w333) -> (x != 0?=w331:bool)
              n225 = Not(x=w332) -> (.not. x?=w330:bool)
              n226 = Equal To 0?(x=w333) -> (x = 0?=w328:bool)
              n227 = And(x=w331, y=w330) -> (x .and. y?=w329:bool)
              n228 = Or(x=w328, y=w329) -> (x .or. y?=w327:bool)
              n229 = Select(t=w333, s=w328, f=w337) -> (s? t:f=w335:i32)
              n230 = property on="XY-Graph" class="XYGraph (strikt)"("Active Plot"=w334, "Plot.Visible?"=w327, "Plot.YScaleIdx"=w333, "Plot.Line Style"=w335) -> ("Plot.Plot Color"=w336:u32)  [unwired: 2 in, 2 out]
              n231 = case shown="True" w338 {
                tunnel: w336 -> [_ w344]
                tunnel: [w341 w343] -> w340
                tunnel: w339 -> [w341 w342]
                frame False {
                }
                frame True {
                  n232 = Insert Into Array(array=w342, new element=w344) -> (w343:u32[])  [unwired: 1 in]
                }
              }
            }
            n233 = for {
              shift-right: [w326] -> _
              shift-left: w313 -> [w323]
              tunnel: w316 -> [w324] mode=indexing
              tunnel: w315 -> [w325]
              tunnel: w314 -> [w322]
              shift-right: [w321] -> _
              shift-left: w313 -> [w320]
              w319 = "\t"
              n234 = Match Pattern(string=w322, regular expression=w319, offset (0)=w320) -> (offset past match=w321:i32)  [unwired: 3 out]
              n235 = Match Pattern(string=w325, regular expression=w319, offset (0)=w323) -> (offset past match=w326:i32)  [unwired: 3 out]
              n236 = property on="Fahrzeugdaten" class="Str"("Text.Selection Start"=w320, "Text.Selection End"=w321, "Text.FontColor"=w324) -> ()  [unwired: 2 in, 2 out]
              n237 = property on="Ergebnis" class="Str"("Text.Selection Start"=w323, "Text.Selection End"=w326, "Text.FontColor"=w324) -> ()  [unwired: 2 in, 2 out]
            }
          }
        }
        n238 = disable-structure shown="Deaktiviert" {
          disable-tunnel: w108 -> [w249 _]
          disable-tunnel: w109 -> [w248 _]
          frame Disabled {
            n239 = flat-sequence {
              tunnel: w249 -> [w254]
              tunnel: w248 -> [w252]
              frame #0 {
                n240 = property on="XY-Graph" class="XYGraph (strikt)"("CrsrList"=T4 [{"Name"="Cursor", "Color"=0, "Style"=2, "Point Style"=0, "Name Visible"=FALSE, "Allow Drag"=TRUE, "Cursor Mode"=2, "Plot"=-1, "Index"=0, "Position"={"X"=0.0, "Y"=0.0}, "X Scale"=0, "Y Scale"=0, "Watch Plots"=[0, 1], "Watch All Plots"=FALSE, "Plot Area"=0, "Label Offset"={"X"=0.0, "Y"=0.0}}] ("Cursor-Liste")) -> ()  [unwired: 2 in, 2 out]
              }
              frame #1 {
                n241 = for {
                  N: w252 -> [_]
                  tunnel: [w255] -> w251 mode=indexing
                  i -> [w255]
                }
                n242 = property on="XY-Graph" class="XYGraph (strikt)"("Active Cursor"=0, "Cursor.Cursor Index"=w254, "Cursor.WatchPlots"=w251) -> ()  [unwired: 2 in, 2 out]
              }
            }
          }
          frame Enabled {
          }
        }
        "Ergebnis" <- w188
        "Fahrzeugdaten" <- w187
      }
      event "Speichern": Value Change {
        n243 = event-data() -> ("OldVal"=w394:bool)  [unwired: 1 in, 5 out]
        n244 = local write "Speichern"(w394) -> ()
        n245 = control-ref of="Datenspeicher"() -> (w393:refnum<vi>)
        n246 = call "savecluster_V0.01.vi"("Datenspeicher 2"=w393) -> ()  [unwired: 2 in]
      }
      event "Stopp": Value Change {
        n247 = event-data() -> ("OldVal"=w395:bool, "NewVal"=w396:bool)  [unwired: 1 in, 4 out]
        n248 = local write "Stopp"(w395) -> ()
      }
      event "Legende": Value Change {
        n249 = event-data() -> ()  [unwired: 1 in, 6 out]
        n250 = local read "XY-Graph"() -> (w400:cluster{dbl[], dbl[]}[])
        n251 = Array Size(array=w400) -> (size(s)=w399:i32)
        n252 = Max & Min(x=w399, y=2) -> (max(x,y)=w397:i32)  [unwired: 1 out]
        n253 = property on="XY-Graph" class="XYGraph (strikt)"("Legend Visible"="Legende", "LegNumRows"=w397) -> ()  [unwired: 2 in, 2 out]
      }
    }
  }
  n254 = property on="XY-Graph" class="XYGraph (strikt)"("Legend Visible"=TRUE, "LegNumRows"=2) -> ()  [unwired: 2 in, 2 out]
  n255 = property on="Fensterbereich" class="Bereich"("Origin"=T3 {"Horizontal"=8, "Vertical"=6}) -> ()  [unwired: 2 in, 2 out]
  n256 = property on="Fensterbereich" class="Bereich"("Origin"=T3 {"Horizontal"=8, "Vertical"=6}) -> ()  [unwired: 2 in, 2 out]
  n257 = property on="Ergebnis" class="Str"("Value"=w12) -> ()  [unwired: 2 in, 2 out]
  n258 = property on="Pmax" class="Str"("Value"=w12) -> ()  [unwired: 2 in, 2 out]
  n259 = property on="Fahrzeugdaten" class="Str"("Value"=w12) -> ()  [unwired: 2 in, 2 out]
  n260 = property on="Datum, Zeit" class="Str"("Value"=w12) -> ()  [unwired: 2 in, 2 out]
  n261 = property on="Gl. Mittelwert" class="DigWert (strikt)"("DisabledEnum"=w2) -> ()  [unwired: 2 in, 2 out]
  n262 = property on="Differenzenquotient" class="DigWert (strikt)"("DisabledEnum"=w2) -> ()  [unwired: 2 in, 2 out]
  n263 = Bundle(w8, w8) -> (w6:cluster{dbl[], dbl[]})  [unwired: 1 in]
  n264 = Bundle(w8, w8) -> (w5:cluster{dbl[], dbl[]})  [unwired: 1 in]
  n265 = case shown="True" "Berechnen" {
    selector: "Berechnen" -> [_ w405]
    frame False {
    }
    frame True {
      n266 = property on="Berechnen" class="Bool. (strikt)"("Value"=w405, "DisabledEnum"=T5."Enabled" ("Deaktiviert")) -> (error out=w402:errorcluster)  [unwired: 2 in, 1 out]
      n267 = property on="Öffnen" class="Bool. (strikt)"(error in=w402, "Val(Sgnl)"=TRUE ("Wert (signalisierend)")) -> ()  [unwired: 1 in, 2 out]
    }
  }
  n268 = property on="Berechnen" class="Bool. (strikt)"("DisabledEnum"=w4) -> ()  [unwired: 2 in, 2 out]
  n269 = property on="Überlagern" class="Bool. (strikt)"("DisabledEnum"=w4) -> ()  [unwired: 2 in, 2 out]
  n270 = property on="Speichern" class="Bool. (strikt)"("DisabledEnum"=w4) -> ()  [unwired: 2 in, 2 out]
  n271 = property on="Drucken" class="Bool. (strikt)"("DisabledEnum"=w4) -> ()  [unwired: 2 in, 2 out]
  n272 = Build Array(w6, w5) -> (w7:cluster{dbl[], dbl[]}[])
  n273 = property on="XY-Graph" class="XYGraph (strikt)"("Value"=w7) -> ()  [unwired: 2 in, 2 out]
